vi "Configure Channel.vi"(7 "Chan Parameters":T1={"Channel"=1, "Chan State"=TRUE, "Chan Sync Source"=0, "Chan Gate Logic"=enum."Disabled", "Chan Mode"=enum."Normal", "Chan Wait #"=0, "Chan Delay"=0.01, "Chan Width"=0.01, "Chan Burst #"=10, "Chan DC On"=10, "Chan DC Off"=10, "Chan Polarity"=FALSE, "Chan MUX Value"=-1, "Chan Level Out"=enum."Adjustable", "Chan Lev Adjust"=5.0, "Chan Gate Mode"=enum."Disabled"} {"Chan Sync Source" items=["System (To)", "Channel A", "Channel B", "Channel C", "Channel D", "Channel E", "Channel F", "Channel G", "Channel H"]; "Chan Width" format="%.3p"; "Chan Delay" format="%.3p"; "Chan Lev Adjust" format="%.3p"; "Channel" items=["Channel A"=1, "Channel B"=2, "Channel C"=3, "Channel D"=4, "Channel E"=5, "Channel F"=6, "Channel G"=7, "Channel H"=8]}, 8 "error in (no error)":errorcluster, 11 "VISA resource name":refnum<visa-resource-name>) -> (0 "error out":errorcluster, 3 "VISA resource name out":refnum<visa-resource-name>)   [LabVIEW 2013]
doc: "This VI demonstrates how to use the \"All Chan Parameters.ctl\" and individual configuration functions to configure a channel.\n\nThe parameters \"Burst #\", \"Divide #\", and \"Adjustable\" are only updated when operating in the corresponding mode."
uses:
  Channel Parameters.ctl
  Public/Configure/Configure Chan Mode (Normal).vi
  Public/Configure/Configure Chan Mode (Single Shot).vi
  Public/Configure/Configure Chan Mode (Duty Cycle).vi
  Public/Configure/Configure Chan Mode (Burst).vi
  Berkeley Nucleonics 500 Series.lvlib
panel:
  # "The parameters \"Burst #\", \"DC On\", \"DC Off\", and \"Adjustable\" are only updated when operating in the corresponding mode."
  # "Input"
  # "Normal\nSingle\nBurst"
  # "Burst"
  # "Duty Cycle"
  # "Output"
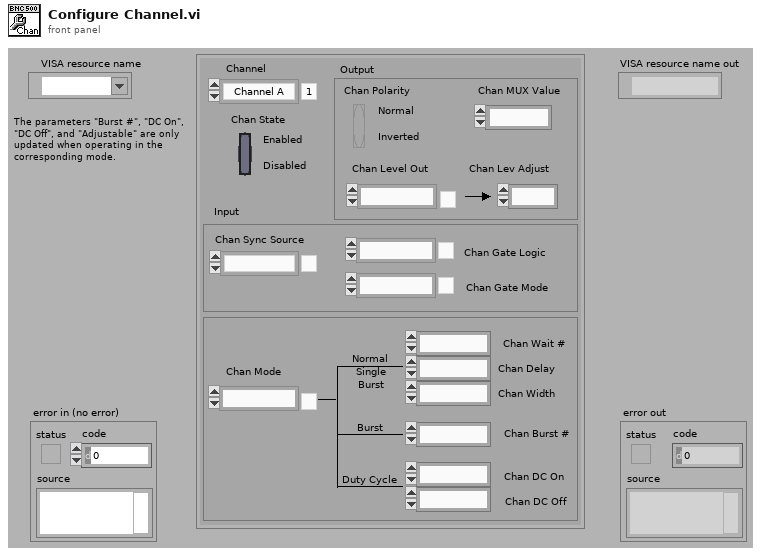
[diagram p1: front panel]
types:
  T1 = typedef "Channel Parameters.ctl" = cluster{"Channel":i32, "Chan State":bool, "Chan Sync Source":i32, "Chan Gate Logic":enum16{"Disabled", "Low", "High"}, "Chan Mode":enum16{"Normal", "Single", "Burst", "Duty Cycle"}, "Chan Wait #":i32, "Chan Delay":dbl, "Chan Width":dbl, "Chan Burst #":i32, "Chan DC On":i32, "Chan DC Off":i32, "Chan Polarity":bool, "Chan MUX Value":i32, "Chan Level Out":enum16{"TTL", "Adjustable", "35 Volt", "Optical"}, "Chan Lev Adjust":dbl, "Chan Gate Mode":enum16{"Disabled", "Pulse Inhibit", "Output Inhibit"}}
  T2 = enum16{"Disabled", "Pulse Inhibit", "Output Inhibit"}
  T3 = enum16{"Normal", "Single", "Burst", "Duty Cycle"}
  T4 = enum16{"TTL", "Adjustable", "35 Volt", "Optical"}
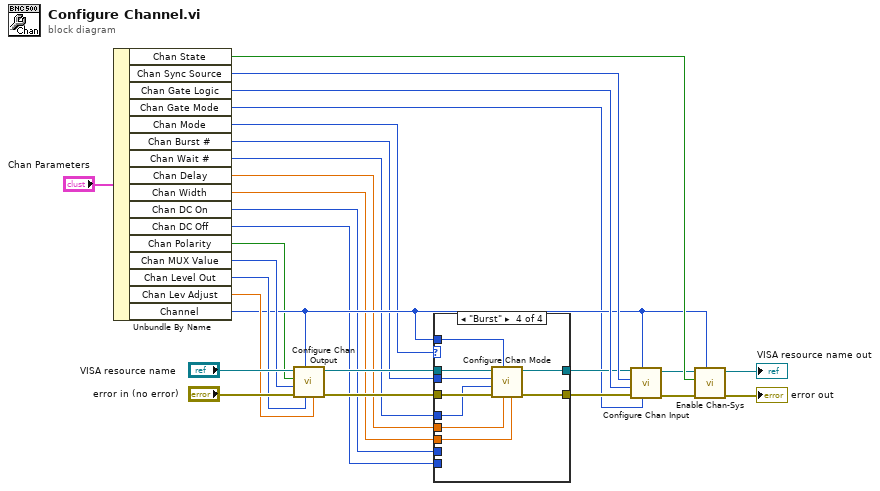
[diagram p0: block diagram]
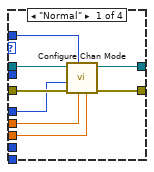
[diagram p2: hidden frame]
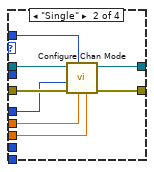
[diagram p3: hidden frame]
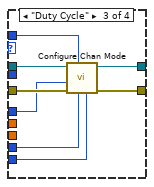
[diagram p4: hidden frame]
diagram:
  n1 = Unbundle By Name("Chan Parameters") -> ("Chan State"=w19:bool, "Chan Sync Source"=w18:i32, "Chan Gate Logic"=w17:enum16{"Disabled", "Low", "High"}, "Chan Gate Mode"=w1:T2, "Chan Mode"=w13:T3, "Chan Burst #"=w3:i32, "Chan Wait #"=w4:i32, "Chan Delay"=w7:dbl, "Chan Width"=w8:dbl, "Chan DC On"=w6:i32, "Chan DC Off"=w5:i32, "Chan Polarity"=w2:bool, "Chan MUX Value"=w22:i32, "Chan Level Out"=w21:T4, "Chan Lev Adjust"=w20:dbl, "Channel"=w14:i32)
  n2 = call "Configure Chan Output.vi"("Adjustable (5 Volts)"=w20, "Level (TTL)"=w21, "Channel (1:Chan A)"=w14, "error in (no error)"="error in (no error)", "MUX Value (-1)"=w22, "Polarity (F:Normal)"=w2, "VISA resource name"="VISA resource name") -> ("error out"=w11:errorcluster, "VISA resource name out"=w12:refnum<visa-resource-name>)  [unwired: 3 in]
  n3 = case shown="\"Burst\"" w13 {
    tunnel: w14 -> [w35 w43 w51 w56]
    tunnel: w12 -> [w34 w42 w50 w60]
    tunnel: w11 -> [w33 w41 w49 w59]
    tunnel: [w32 w40 w48 w58] -> w10
    tunnel: [w31 w39 w47 w57] -> w9
    tunnel: w7 -> [w29 w36 _ w54]
    tunnel: w4 -> [w30 w38 w46 w55]
    tunnel: w8 -> [w28 w37 _ w53]
    tunnel: w6 -> [_ _ w45 _]
    tunnel: w5 -> [_ _ w44 _]
    tunnel: w3 -> [_ _ _ w52]
    frame "Normal" {
      n4 = call-poly "Configure Chan Mode.vi"("Width (10 msec)"=w28, "Delay (10 msec)"=w29, "Channel (1:Chan A)"=w35, "error in (no error)"=w33, "Wait # (0)"=w30, "VISA resource name"=w34) -> ("error out"=w31:errorcluster, "VISA resource name out"=w32:refnum<visa-resource-name>)  [unwired: 4 in]
    }
    frame "Single" {
      n5 = call-poly "Configure Chan Mode.vi"("Width (10 msec)"=w37, "Delay (10 msec)"=w36, "Channel (1:Chan A)"=w43, "error in (no error)"=w41, "Wait # (0)"=w38, "VISA resource name"=w42) -> ("error out"=w39:errorcluster, "VISA resource name out"=w40:refnum<visa-resource-name>)  [unwired: 4 in]
    }
    frame "Duty Cycle" {
      n6 = call-poly "Configure Chan Mode.vi"("Chan DC Off (10)"=w44, "Chan DC On (10)"=w45, "Channel (1:Chan A)"=w51, "error in (no error)"=w49, "Wait # (0)"=w46, "VISA resource name"=w50) -> ("error out"=w47:errorcluster, "VISA resource name out"=w48:refnum<visa-resource-name>)  [unwired: 4 in]
    }
    frame "Burst" {
      n7 = call-poly "Configure Chan Mode.vi"("Width (10 msec)"=w53, "Delay (10 msec)"=w54, "Channel (1:Chan A)"=w56, "error in (no error)"=w59, "Wait # (0)"=w55, "Burst # (10)"=w52, "VISA resource name"=w60) -> ("error out"=w57:errorcluster, "VISA resource name out"=w58:refnum<visa-resource-name>)  [unwired: 3 in]
    }
  }
  n8 = call "Configure Chan Input.vi"("Gate Mode (0:Disabled)"=w1, "Channel (1:Chan A)"=w14, "error in (no error)"=w9, "Gate Logic (0:Disabled)"=w17, "Sync Source (0:To)"=w18, "VISA resource name"=w10) -> ("error out"=w15:errorcluster, "VISA resource name out"=w16:refnum<visa-resource-name>)  [unwired: 4 in]
  n9 = call "Enable Chan-Sys.vi"("Channel (1:Chan A)"=w14, "error in (no error)"=w15, "State (T:Enabled)"=w19, "VISA resource name"=w16) -> ("error out"=→"error out":errorcluster, "VISA resource name out"=→"VISA resource name out":refnum<visa-resource-name>)  [unwired: 6 in]
